vi "Load.vi"(8 "error in (no error)":errorcluster, 10 "JSON":string, 11 "VisionUI in":refnum<class "VisionUI.lvclass">) -> (0 "error out":errorcluster, 3 "VisionUI out":refnum<class "VisionUI.lvclass">)   [LabVIEW 2021, in "VisionUI.lvlib" / "VisionUI.lvclass"]
uses:
  VisionUI.lvclass
  3b109f1e-f283-4af2-9373-7efebe262c1d.vi
  <vilib>/JDP Science/JSONtext/String Subset.vi
  <vilib>/JDP Science/JSONtext/Parsing/Parse Full Path or Item Name.vi
  <vilib>/JDP Science/JSONtext/Next JSON Value.vi
  <vilib>/JDP Science/JSONtext/support/Error Cluster From Code.vi
  <vilib>/JDP Science/JSONtext/Offset/Find Item Locations by Path.vi
  <vilib>/JDP Science/JSONtext/JSON text to Variant.vi
  Vision/Vision/Vision.lvclass
  <vilib>/JDP Science/JSONtext/LVClass Serializer/JSONtext LVClass Serializer.lvclass
  <vilib>/JDP Science/JSONtext/JSONtext.lvlib
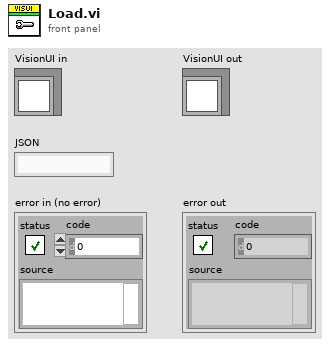
[diagram p1: front panel]
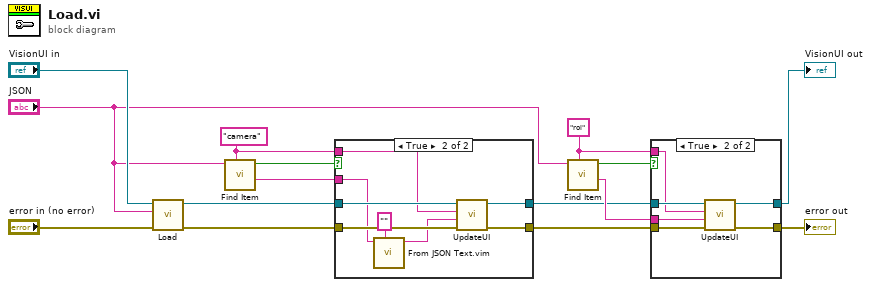
[diagram p0: block diagram]
diagram:
  w8 = "roi" ("$Path or Item Name")
  w10 = "camera" ("$Path or Item Name")
  n1 = call-parent "Load.vi"("error in (no error)"="error in (no error)", "JSON"="JSON", "Vision in"="VisionUI in") -> ("error out"=w12:errorcluster, "Vision out"=w13:refnum<class "VisionUI.lvclass">)  [unwired: 7 in]
  n2 = call <vilib>:"Find Item.vi"("$Path or Item Name"=w10, "JSON"="JSON") -> ("<JSON>"=w1:string, "Found"=w11:bool)  [unwired: 6 in, 2 out]
  n3 = case shown="True" w11 {
    tunnel: w13 -> [w17 w25]
    tunnel: w12 -> [w16 w24]
    tunnel: w10 -> [_ w23]
    tunnel: [w17 w22] -> w6
    tunnel: [w16 w21] -> w4
    tunnel: w1 -> [_ w19]
    frame False {
    }
    frame True {
      n4 = call "From JSON Text.vim"("Data Type and Default Value"="", "JSON"=w19) -> ("Data out"=w18:string)  [unwired: 8 in, 1 out]
      n5 = call "UpdateUI.vi"("error in (no error)"=w24, "Json Data"=w18, "Type"=w23, "VisionUI in"=w25) -> ("error out"=w21:errorcluster, "VisionUI out"=w22:refnum<class "VisionUI.lvclass">)  [unwired: 6 in]
    }
  }
  n6 = call <vilib>:"Find Item.vi"("$Path or Item Name"=w8, "JSON"="JSON") -> ("<JSON>"=w7:string, "Found"=w9:bool)  [unwired: 6 in, 2 out]
  n7 = case shown="True" w9 {
    tunnel: w6 -> [w27 w33]
    tunnel: w4 -> [w26 w32]
    tunnel: w8 -> [_ w31]
    tunnel: w7 -> [_ w30]
    tunnel: [w27 w29] -> w3
    tunnel: [w26 w28] -> w2
    frame False {
    }
    frame True {
      n8 = call "UpdateUI.vi"("error in (no error)"=w32, "Json Data"=w30, "Type"=w31, "VisionUI in"=w33) -> ("error out"=w28:errorcluster, "VisionUI out"=w29:refnum<class "VisionUI.lvclass">)  [unwired: 6 in]
    }
  }
  "error out" <- w2
  "VisionUI out" <- w3
